vi "Encode-Decode Parameters (core).vi"(9 "Payload size - bytes":i32=16, 10 "Parameters":T2(array[cluster])=[{"start index"=0, "size"=64, "encoding"=0, "signed"=TRUE, "scale multiplier"=1.0, "scale offset"=0.0}, {"start index"=64, "size"=64, "encoding"=0, "signed"=TRUE, "scale multiplier"=1.0, "scale offset"=0.0}] {"encoding" items=["BNR", "BCD", "Discrete", "Signed_32", "Signed_64", "Float_32", "Float_64", "Opaque"]}, 11 "Values in":dbl[](array[numeric])) -> (2 "Result array out":bool[](array[boolean]), 3 "Values out":dbl[](array[numeric]))   [LabVIEW 2020]
uses:
  Shared/Encoding (Arinc664).ctl
  Engine/Implementation/Rx UDP Execution Unit/Rx UDP Execution Unit.lvclass
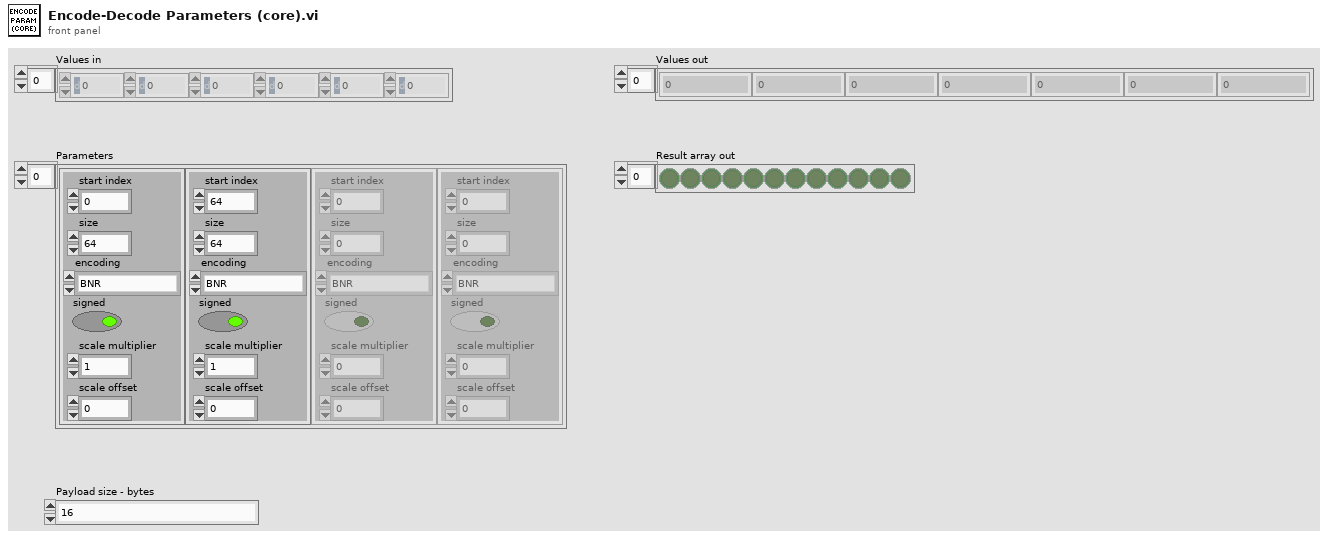
[diagram p1: front panel]
types:
  T1 = typedef "Encoding (Arinc664).ctl" = u16
  T2 = cluster{"start index":i32, "size":i32, "encoding":T1, "signed":bool, "scale multiplier":dbl, "scale offset":dbl}[]
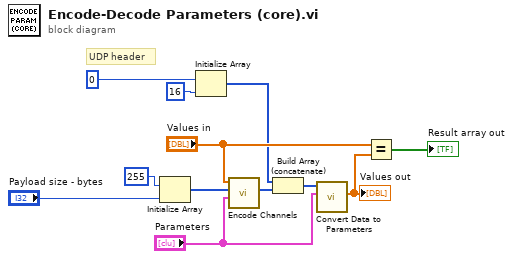
[diagram p0: block diagram]
diagram:
  # "UDP header"
  n1 = Initialize Array(255 ("dimension size"), "Payload size - bytes") -> (w10:i32[])
  n2 = Initialize Array(u8 0 ("element"), 16 ("dimension size")) -> (w5:u8[])
  n3 = call "Encode Channels.vi"("Parameters"="Parameters", "Data in"=w10, "Values in"="Values in") -> ("Data out"=w2:u8[])  [unwired: 6 in, 2 out]
  n4 = Build Array (concatenate)(w5, w2) -> (w1:u8[])
  n5 = call "Convert Data to Parameters.vi"("Parameters"="Parameters", "Message Buffer in"=w1) -> ("Array"=w7:dbl[])  [unwired: 8 in, 1 out]
  "Values out" <- w7
  n6 = Equal?(x="Values in", y=w7) -> (x = y?=→"Result array out":bool[])
